vi "setDomainReadType.vi"(8 "error in (no error)":errorcluster, 10 "SampleType in":T1 items=["daqSampleTypeInvalid", "daqSampleTypeFloat32", "daqSampleTypeFloat64", "daqSampleTypeUInt8", "daqSampleTypeInt8", "daqSampleTypeUInt16", "daqSampleTypeInt16", "daqSampleTypeUInt32", "daqSampleTypeInt32", "daqSampleTypeUInt64", "daqSampleTypeInt64", "daqSampleTypeRangeInt64", "daqSampleTypeComplexFloat32", "daqSampleTypeComplexFloat64", "daqSampleTypeBinary", "daqSampleTypeString", "daqSampleTypeStruct", "daqSampleTypeNull", "daqSampleType_count"], 11 "IMultiReaderBuilder in":refnum<class "IMultiReaderBuilder.lvclass">) -> (0 "error out":errorcluster, 3 "IMultiReaderBuilder out":refnum<class "IMultiReaderBuilder.lvclass">)   [LabVIEW 2022 SP3, in "openDAQ.lvlib" / "IBaseObject.lvlib" / "IMultiReaderBuilder.lvlib" / "IMultiReaderBuilder.lvclass"]
uses:
  <instrlib>/openDAQ/Public/Classes/IMultiReaderBuilder/IMultiReaderBuilder.lvclass
  C:/Program Files (x86)/National Instruments/LabVIEW 2022/instr.lib/openDAQ/Public/Classes/IBaseObject/IBaseObject.lvclass
  <instrlib>/openDAQ/Public/TypeDef/daqSampleType.ctl
  <instrlib>/openDAQ/Public/Classes/IBaseObject/IBaseObject.lvclass/IBaseObject.ctl
  <instrlib>/openDAQ/Public/Classes/IBaseObject/Accessor/Read reference.vi
  <instrlib>/openDAQ/Public/Classes/IBaseObject/Accessor/Write reference.vi
  <instrlib>/openDAQ/Binaries/Windows/x86/copendaq32.dll
  <instrlib>/openDAQ/openDAQ.lvlib
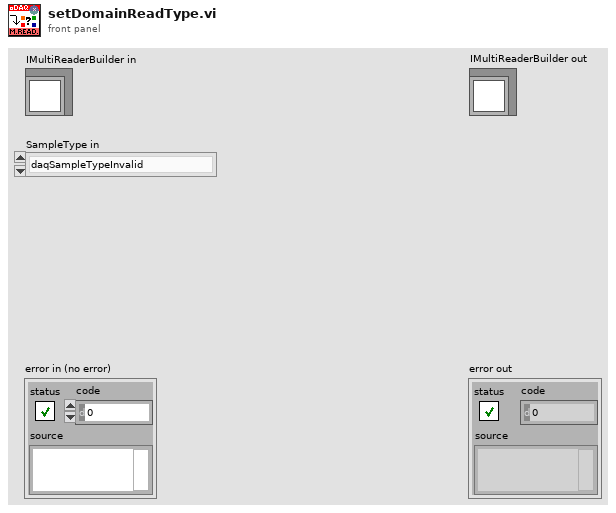
[diagram p1: front panel]
types:
  T1 = typedef "openDAQ.lvlib/daqSampleType.ctl" = u16
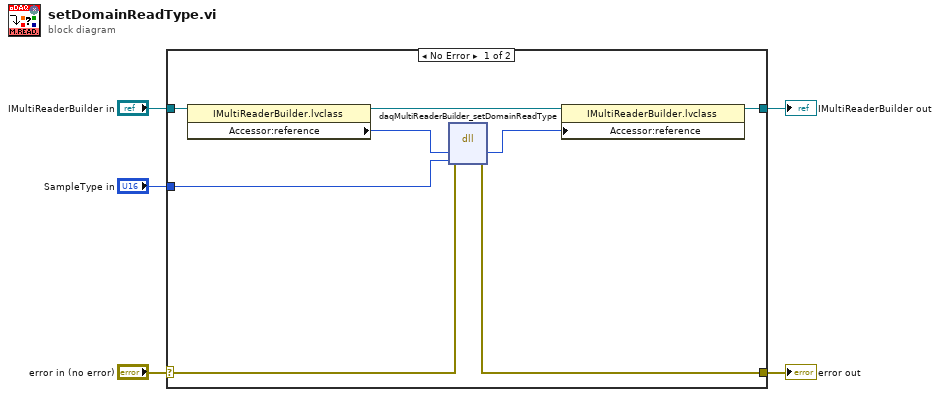
[diagram p0: block diagram]
diagram:
  n1 = case shown="No Error" "error in (no error)" {
    selector: "error in (no error)" -> [w12 w15]
    tunnel: [w11 w15] -> w4
    tunnel: [w9 w14] -> w2
    tunnel: "IMultiReaderBuilder in" -> [w13 w14]
    tunnel: "SampleType in" -> [w6 _]
    frame No Error {
      n2 = property class="IMultiReaderBuilder.lvclass"(reference=w13) -> (reference out=w10:refnum<class "IMultiReaderBuilder.lvclass">, "Accessor:reference"=w8:i64)  [unwired: 1 in, 1 out]
      n3 = dll-call lib="C:/Program Files (x86)/National Instruments/LabVIEW 2022/instr.lib/openDAQ/Binaries/Windows/x86/copendaq*.*" fn="daqMultiReaderBuilder_setDomainReadType"(error in=w12, "builder"=w8, "readType"=w6) -> (error out=w11:errorcluster, "builder"=w7:i64)  [unwired: 4 in, 1 out]
      n4 = property class="IMultiReaderBuilder.lvclass"(reference=w10, "Accessor:reference"=w7) -> (reference out=w9:refnum<class "IMultiReaderBuilder.lvclass">)  [unwired: 1 in, 1 out]
    }
    frame Error {
    }
  }
  "error out" <- w4
  "IMultiReaderBuilder out" <- w2
